vi "Scanner List Item to Scanner Name.vi"(1 "Scanner List Item":T1) -> (0 "Scanner Name":string)   [LabVIEW 2017, in "Scan Driver.lvclass"]
uses:
  Scan Driver.lvclass
  Scanner List.ctl
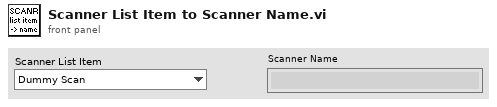
[diagram p1: front panel]
types:
  T1 = typedef "Scan Driver.lvclass/Scanner List.ctl" = enum16{"Dummy Scan", "Analog Output Scan", "Function Gen Scan", "Magnetic Field Lakeshore", "Magnetic Field Lakeshore Continuous", "Magnetic Field Oxford", "Magnetic Field Oxford Continuous", "Magna Current Scan", "Magna Voltage Scan", "Microwave Freq Scan", "Pulse Gen Scan", "Pulse Gen Basic Scan", "Translation Stage Dual", "Translation Stage Coarse", "Translation Stage Fine", "Wavelength Triax 550", "Wavelength Digikröm", "Wavelength ActiveX", "None"}
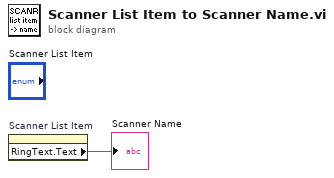
[diagram p0: block diagram]
diagram:
  n1 = property on="Scanner List Item" class="Enum (strict)"() -> ("RingText.Text"=→"Scanner Name":string)  [unwired: 2 in, 2 out]
